vi "Broadcast Response.vi"(8 "error in (no error)":errorcluster, 9 "Acquired Result.lvclass":refnum<class "Acquired Result.lvclass">, 10 "Topic":string, 11 "Measure Object in":refnum<class "Communications.lvclass">) -> (0 "error out":errorcluster, 3 "Measure Object out":refnum<class "Communications.lvclass">)   [LabVIEW 2016, in "Communications.lvclass"]
uses:
  Communications.lvclass
  Results/Acquired Result/Acquired Result.lvclass
  Template Module/Template Module.lvclass
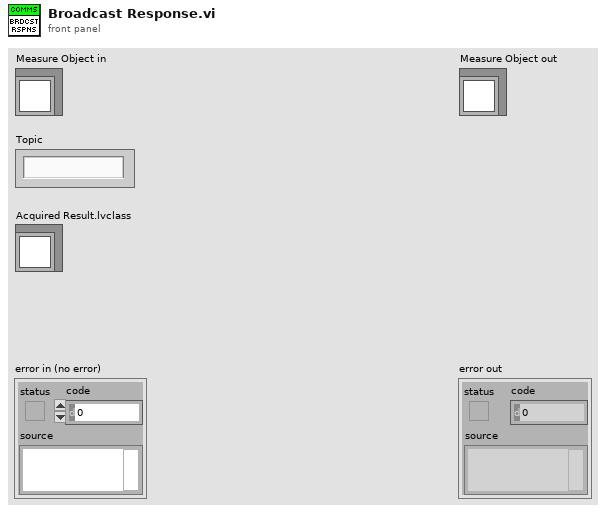
[diagram p1: front panel]
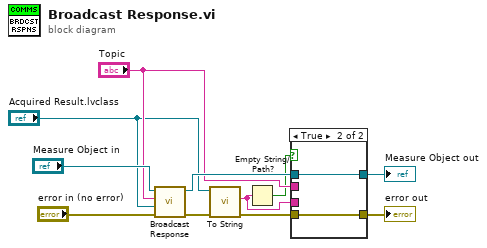
[diagram p0: block diagram]
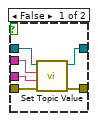
[diagram p2: hidden frame]
diagram:
  n1 = call-parent "Broadcast Response.vi"("error in (no error)"="error in (no error)", "Acquired Result.lvclass"="Acquired Result.lvclass", "Topic"="Topic", "Measure Object in"="Measure Object in") -> ("error out"=w4:errorcluster, "Measure Object out"=w9:refnum<class "Communications.lvclass">)  [unwired: 6 in]
  n2 = call-dynamic "To String.vi"("error in (no error)"=w4, "Acquired Result in"="Acquired Result.lvclass") -> ("error out"=w5:errorcluster, "String"=w2:string)  [unwired: 7 in, 1 out]
  n3 = Empty String/Path?(string/path=w2) -> (empty?=w1:bool)
  n4 = case shown="True" w1 {
    tunnel: w9 -> [w17 w19]
    tunnel: [w16 w19] -> w8
    tunnel: "Topic" -> [w15 _]
    tunnel: w5 -> [w14 w18]
    tunnel: [w13 w18] -> w3
    tunnel: w2 -> [w12 _]
    frame False {
      n5 = call-dynamic "Set Topic Value.vi"("error in (no error)"=w14, "Value"=w12, "Topic"=w15, "Communications in"=w17) -> ("error out"=w13:errorcluster, "Communications out"=w16:refnum<class "Communications.lvclass">)  [unwired: 5 in, 1 out]
    }
    frame True {
    }
  }
  "error out" <- w3
  "Measure Object out" <- w8
